vi "read config.vi"(7 "Section":string, 8 "error in (no error) 2":errorcluster, 9 "Default value":string, 10 "Key":string, 11 "refnum":T1) -> (0 "error out":errorcluster, 1 "value":string, 3 "refnum out":T1)   [LabVIEW 2015]
uses:
  <vilib>/Utility/config.llb/Config Data RefNum.ctl
  <vilib>/Utility/config.llb/Read Key (String).vi
  <vilib>/Utility/config.llb/Write Key (String).vi
  <vilib>/Utility/config.llb/NI_LVConfig.lvlib
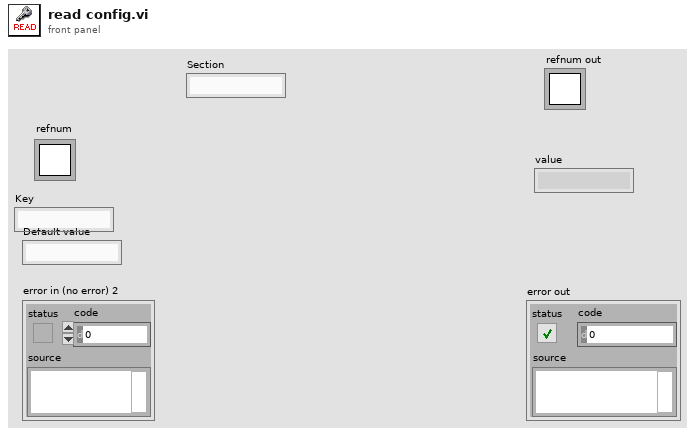
[diagram p1: front panel]
types:
  T1 = typedef "NI_LVConfig.lvlib/Config Data RefNum.ctl" = refnum<k1>
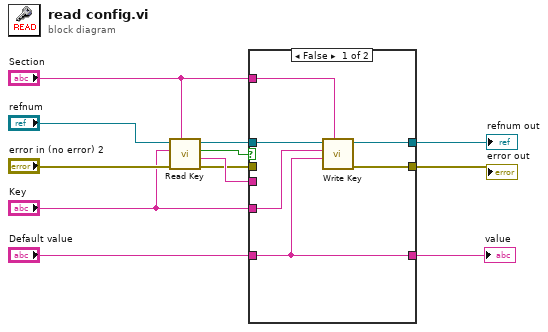
[diagram p0: block diagram]
diagram:
  n1 = call-poly <vilib>:"Read Key.vi"("section"="Section", "error in (no error)"="error in (no error) 2", "key"="Key", "refnum"="refnum") -> ("error out"=w5:errorcluster, "value"=w11:string, "found?"=w1:bool, "refnum out"=w4:T1)  [unwired: 4 in]
  n2 = case shown="False" w1 {
    tunnel: "Section" -> [w18 _]
    tunnel: "Key" -> [w17 _]
    tunnel: w4 -> [w16 w21]
    tunnel: w5 -> [_ w20]
    tunnel: "Default value" -> [w13 _]
    tunnel: [w15 w21] -> w9
    tunnel: [w14 w20] -> w10
    tunnel: w11 -> [_ w19]
    tunnel: [w13 w19] -> w12
    frame False {
      n3 = call-poly <vilib>:"Write Key.vi"("section"=w18, "value"=w13, "key"=w17, "refnum"=w16) -> ("error out"=w14:errorcluster, "refnum out"=w15:T1)  [unwired: 5 in, 1 out]
    }
    frame True {
    }
  }
  "refnum out" <- w9
  "error out" <- w10
  "value" <- w12
